vi "set_headers.vi"(6 "header_value []":cluster{"header":string, "value":string}[](array[cluster]), 8 "error in (no error)":errorcluster, 11 "client_handle in":T1) -> (0 "error out":errorcluster, 3 "client_handle out":T1)   [LabVIEW 2015, in "lv-dropbox.lvlib"]
uses:
  lv-dropbox.lvlib
  <vilib>/httpClient/ClientHandle.ctl
  <vilib>/httpClient/LabVIEWHTTPClient.lvlib
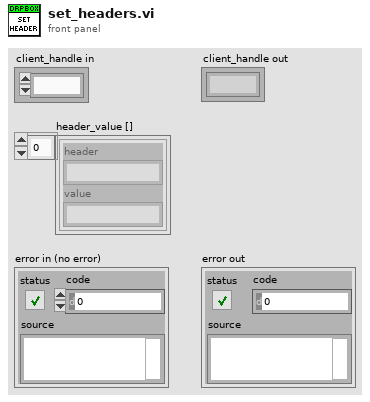
[diagram p1: front panel]
types:
  T1 = typedef "LabVIEWHTTPClient.lvlib/ClientHandle.ctl" = refnum<k1>
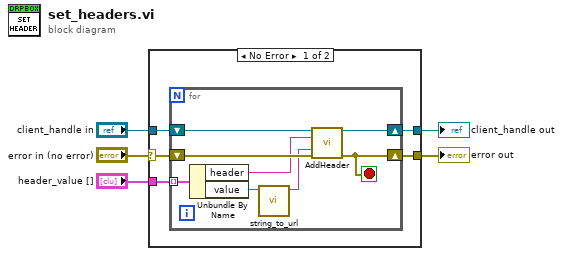
[diagram p0: block diagram]
diagram:
  n1 = case shown="No Error" "error in (no error)" {
    selector: "error in (no error)" -> [w9 w20]
    tunnel: [w10 w19] -> w5
    tunnel: [w8 w20] -> w3
    tunnel: "client_handle in" -> [w7 w19]
    tunnel: "header_value []" -> [w6 _]
    frame No Error {
      n2 = for {
        shift-right: [w17] -> w10
        shift-left: w7 -> [w18]
        shift-right: [w15] -> w8
        shift-left: w9 -> [w16]
        tunnel: w6 -> [w14] mode=indexing
        stop <- w15 stop-if-true
        n3 = Unbundle By Name(w14) -> ("header"=w13:string, "value"=w12:string)
        n4 = call "string_to_url.vi"("string"=w12) -> ("url"=w11:string)  [unwired: 10 in]
        n5 = call <vilib>:"AddHeader.vi"("client handle"=w18, "header"=w13, "value"=w11, "error in (no error)"=w16) -> ("client handle out"=w17:T1, "error out"=w15:errorcluster)  [unwired: 10 in]
      }
    }
    frame Error {
    }
  }
  "client_handle out" <- w5
  "error out" <- w3
